vi "Set DB Connection Parameters.vi"(8 "error in (no error)":errorcluster, 11 "database in":refnum<class "database.lvclass">) -> (0 "error out":errorcluster, 3 "database out":refnum<class "database.lvclass">)   [LabVIEW 2018, in "database.lvclass"]
uses:
  database.lvclass
  database.lvclass/database.ctl
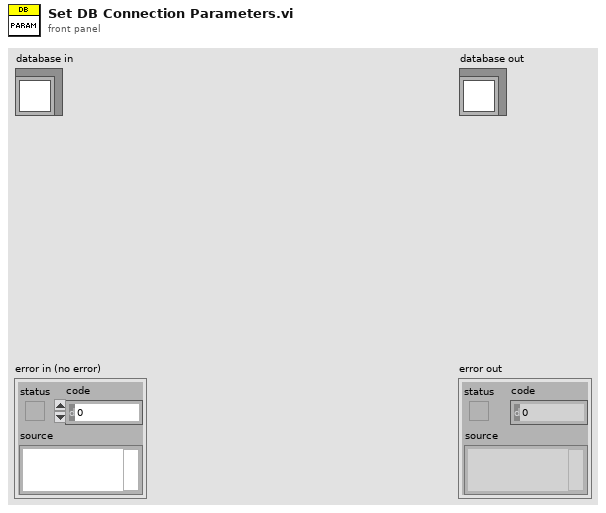
[diagram p1: front panel]
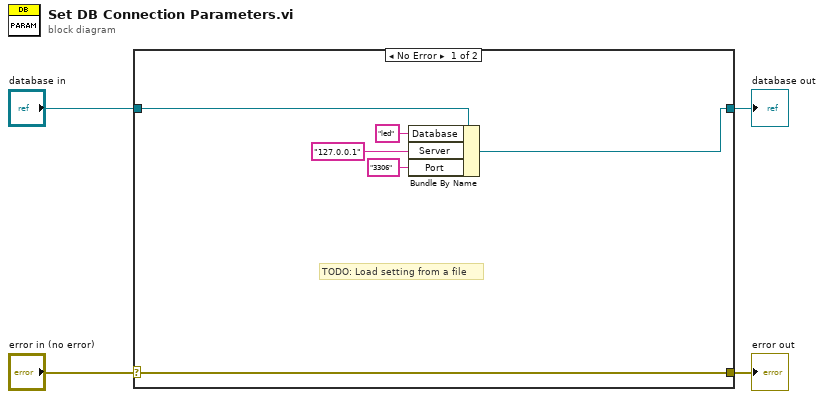
[diagram p0: block diagram]
diagram:
  n1 = case shown="No Error" "error in (no error)" {
    selector: "error in (no error)" -> [w10 w12]
    tunnel: [w10 w12] -> w3
    tunnel: [w8 w11] -> w1
    tunnel: "database in" -> [w9 w11]
    frame No Error {
      # "TODO: Load setting from a file"
      n2 = Bundle By Name(cluster=w9, "Database"="led", "Server"="127.0.0.1" ("Database"), "Port"="3306") -> (w8:refnum<class "database.lvclass">)
    }
    frame Error {
    }
  }
  "error out" <- w3
  "database out" <- w1
